vi "GetSerializableDataCommon.vi"(8 "error in (no error)":errorcluster, 9 "Options":T1, 10 "Data (FromParent)":T3, 11 "SerializableData":variant) -> (0 "error out":errorcluster, 2 "Data":T3)   [LabVIEW 2019, in "BlueSerialization.lvlib" / "BlueSerializer.lvclass"]
uses:
  BlueSerializer.lvclass
  GetSerializableDataCluster.ctl
  GetSerializableDataAction.ctl
  GetSerializableDataClusterClass.ctl
  SerializableDataGetDataAction.ctl
  ClassNameAndVersion.ctl
  <vilib>/Utility/EditLVLibs/LibVersion.ctl
  SerializeOptionsPayload.ctl
  SerializeOptions.ctl
  ClassNameCacheMap.ctl
  ClassNameObj.ctl
  <vilib>/Utility/Data Type/Get Type Information.vi
  <vilib>/Utility/Data Type/Get Cluster Information.vi
  <vilib>/Utility/EditLVLibs/Edit LVLibs.lvlib
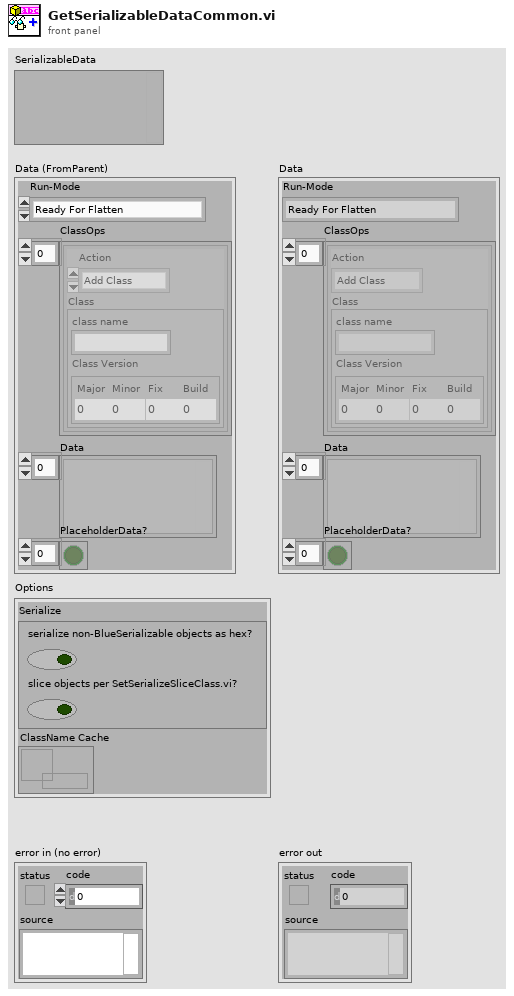
[diagram p1: front panel]
types:
  T1 = typedef "BlueSerialization.lvlib/BlueSerializer.lvclass/SerializeOptionsPayload.ctl" = cluster{"Serialize":T2, "ClassName Cache":refnum<data-value>}
  T2 = typedef "BlueSerialization.lvlib/BlueSerializer.lvclass/SerializeOptions.ctl" = cluster{"serialize non-BlueSerializable objects as hex?":bool, "slice objects per SetSerializeSliceClass.vi?":bool}
  T3 = typedef "BlueSerialization.lvlib/BlueSerializer.lvclass/GetSerializableDataCluster.ctl" = cluster{"Run-Mode":T4, "ClassOps":T5[], "Data":variant[], "PlaceholderData?":bool[]}
  T4 = typedef "BlueSerialization.lvlib/BlueSerializer.lvclass/GetSerializableDataAction.ctl" = enum16{"Ready For Flatten", "Unmodified Data Access"}
  T5 = typedef "BlueSerialization.lvlib/BlueSerializer.lvclass/GetSerializableDataClusterClass.ctl" = cluster{"Action":T6, "Class":T7}
  T6 = typedef "BlueSerialization.lvlib/BlueSerializer.lvclass/SerializableDataGetDataAction.ctl" = enum16{"Add Class", "Drop Class"}
  T7 = typedef "BlueSerialization.lvlib/BlueSerializer.lvclass/ClassNameAndVersion.ctl" = cluster{"class name":string, "Class Version":T8}
  T8 = typedef "Edit LVLibs.lvlib/LibVersion.ctl" = cluster{"Major":u16, "Minor":u16, "Fix":u16, "Build":u16}
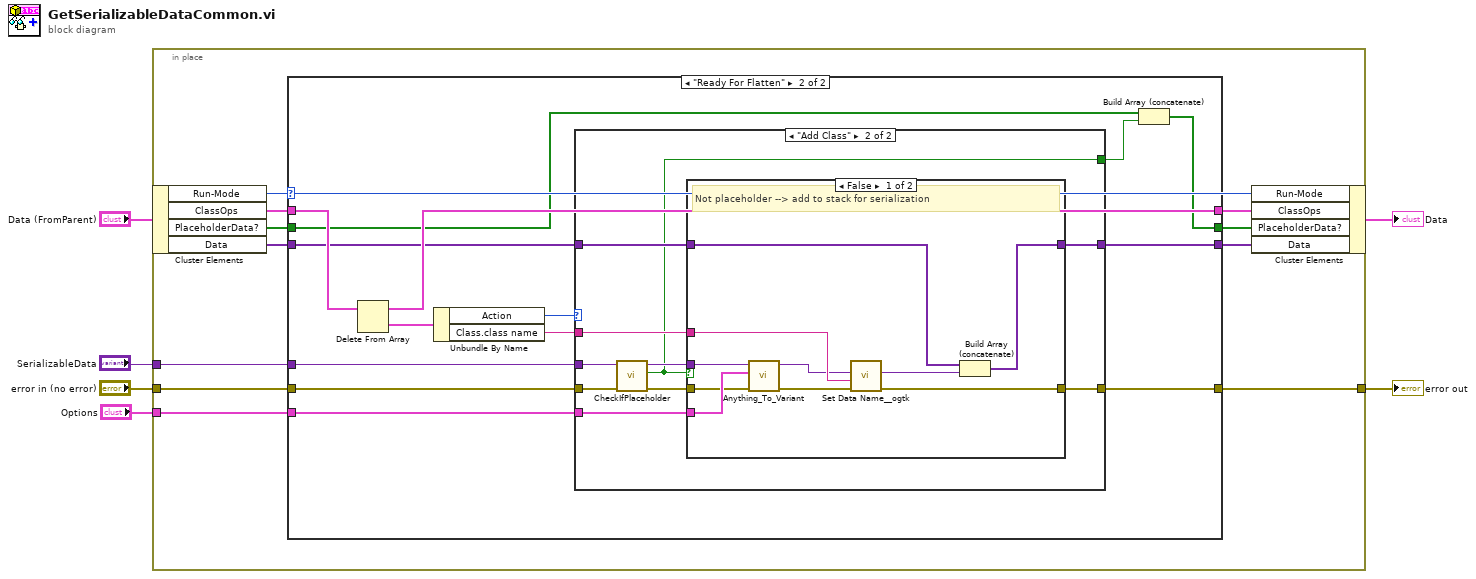
[diagram p0: block diagram]
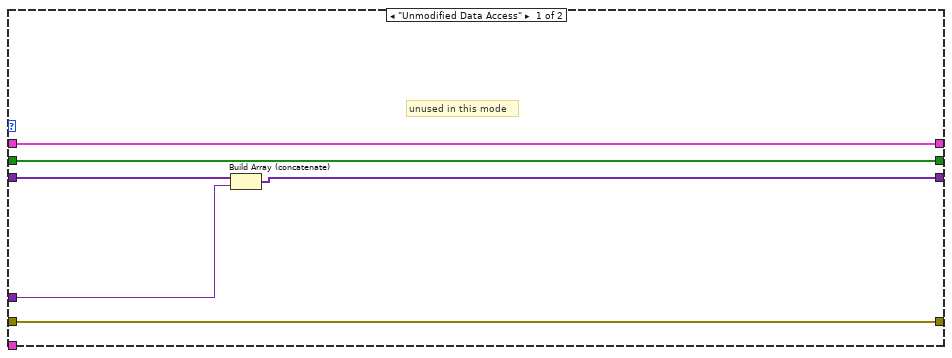
[diagram p2: hidden frame]
diagram:
  n1 = in-place {
    in-place-border: "SerializableData" -> [w13]
    in-place-border: "error in (no error)" -> [w12]
    in-place-border: [w11] -> w2
    in-place-border: "Options" -> [w10]
    n2 = in-place-cluster #1("Data (FromParent)") -> ("Run-Mode"=w9:T4, "ClassOps"=w17:T5[], "PlaceholderData?"=w8:bool[], "Data"=w15:variant[])
    n3 = case shown="\"Ready For Flatten\"" w9 {
      tunnel: w17 -> [w23 w37]
      tunnel: [w23 w36] -> w16
      tunnel: w15 -> [w22 w35]
      tunnel: [w20 w34] -> w14
      tunnel: w13 -> [w21 w33]
      tunnel: w12 -> [w19 w32]
      tunnel: [w19 w31] -> w11
      tunnel: w10 -> [_ w30]
      tunnel: w8 -> [w18 w25]
      tunnel: [w18 w24] -> w7
      frame "Unmodified Data Access" {
        # "unused in this mode"
        n4 = Build Array (concatenate)(w22, w21) -> (w20:variant[])
      }
      frame "Ready For Flatten" {
        n5 = Delete From Array(array=w37) -> (deleted portion=w29:T5, array with subset deleted=w36:T5[])  [unwired: 2 in]
        n6 = Unbundle By Name(w29) -> ("Action"=w27:T6, "Class.class name"=w28:string)
        n7 = case shown="\"Add Class\"" w27 {
          tunnel: w35 -> [w39 w49]
          tunnel: [w39 w48] -> w34
          tunnel: w33 -> [_ w44]
          tunnel: w32 -> [w38 w43]
          tunnel: [w38 w45] -> w31
          tunnel: w30 -> [_ w47]
          tunnel: w28 -> [_ w46]
          tunnel: [_ w40] -> w26
          frame "Drop Class" {
          }
          frame "Add Class" {
            n8 = call "CheckIfPlaceholder.vi"("error in (no error)"=w43, "Data"=w44) -> ("error out"=w41:errorcluster, "IsPlacerholder?"=w40:bool, "Data (dup)"=w42:variant)  [unwired: 7 in]
            n9 = case shown="False" w40 {
              tunnel: w49 -> [w59 w60]
              tunnel: [w58 w60] -> w48
              tunnel: w47 -> [w57 _]
              tunnel: w46 -> [w56 _]
              tunnel: [w54 w61] -> w45
              tunnel: w42 -> [w51 _]
              tunnel: w41 -> [w50 w61]
              frame False {
                # "Not placeholder --> add to stack for serialization"
                n10 = call "Anything_To_Variant.vi"("error in (no error)"=w50, "Options"=w57, "Anything"=w51) -> ("error out"=w52:errorcluster, "Serialized Variant"=w53:variant)  [unwired: 7 in]
                n11 = call <userlib>:"Set Data Name__ogtk.vi"("error in (no error)"=w52, "Data Name"=w56, "Data"=w53) -> ("error out"=w54:errorcluster, "Renamed Data"=w55:variant)  [unwired: 7 in]
                n12 = Build Array (concatenate)(w59, w55) -> (w58:variant[])
              }
              frame True {
                # "placeholder --> don't serialize it!"
              }
            }
          }
        }
        n13 = Build Array (concatenate)(w25, w26) -> (w24:bool[])
      }
    }
    n14 = in-place-cluster #1("Run-Mode"=w9, "ClassOps"=w16, "PlaceholderData?"=w7, "Data"=w14) -> (→"Data":T3)
  }
  "error out" <- w2
